vi "PALETTE.vi"   [LabVIEW 2020]
uses:
  Typedefs/Frame Size.ctl
  Typedefs/AOL modes.ctl
  Typedefs/Plane Mode.ctl
  User Interface/Visualisation/Functional Imaging Viewer/SubVIs/Experiment header interface/Typedefs/Header parameters cluster-Live imaging.ctl
  Typedefs/AOL Properties Cluster.ctl
  Global Variables/General Globals.vi
  User Interface/Visualisation/Functional Imaging Viewer/xcontrol/Typedefs/Xctl-XY data type definition.ctl
  User Interface/Visualisation/Functional Imaging Viewer/xcontrol/XGrapher.xctl
  User Interface/Visualisation/Functional Imaging Viewer/xcontrol/Typedefs/Xcrtl-Data format definition.ctl
  User Interface/Visualisation/Functional Imaging Viewer/Typedefs/Get-Set-Clear Control.ctl
  User Interface/Visualisation/Functional Imaging Viewer/xcontrol/Typedefs/Xctrl-ROI type enum.ctl
types:
  T1 = typedef "Get-Set-Clear Control.ctl" = enum16{"Get", "Set", "Clear"}
  T2 = typedef "XGrapher.xctl/Xcrtl-Data format definition.ctl" = cluster{"Plot.Plot Name":string, "Data":T3, "Timeline data":T3, "Type":T4, "Points per cycle":u16, "ROI index":u16}
  T3 = typedef "XGrapher.xctl/Xctl-XY data type definition.ctl" = cluster{"X-Axis values":sgl[], "Y-Axis values (s)":sgl[]}
  T4 = typedef "Xctrl-ROI type enum.ctl" = enum16{"POI", "Mini-scan", "Group"}
  T5 = typedef "Header parameters cluster-Live imaging.ctl" = cluster{"Frame Size":T6, "Field of View":dbl, "Zoom":u16, "X centre":dbl, "Y centre":dbl, "DwellTime (us)":dbl, "AOL Z":dbl, "Wavelength (nm)":dbl, "Laser power (%)":u8, "Pockels":dbl, "Back Apperture":dbl, "PMT 1":dbl, "PMT 2":dbl, "# Averaged Frames":u8, "AOL Mode":T7, "Angle (degrees)":dbl, "Plane Mode":T8, "Video length (sec)":dbl, "Frame rate (fps)":u8, "Fill time (us)":dbl}
  T6 = typedef "Frame Size.ctl" = u16
  T7 = typedef "AOL modes.ctl" = enum16{"Raster", "Structural", "Pointing", "Mini Scan", "Alignment"}
  T8 = typedef "Plane Mode.ctl" = u16
  T9 = typedef "AOL Properties Cluster.ctl" = cluster{"AOD 1 thickness (mm)":dbl, "AOD 2 thickness (mm)":dbl, "AOD 3 thickness (mm)":dbl, "AOD 4 thickness (mm)":dbl, "AOD 5 thickness (mm)":dbl, "AOD 6 thickness (mm)":dbl, "AOD 1-2 separation (mm)":dbl, "AOD 2-3 separation (mm)":dbl, "AOD 3-4 separation (mm)":dbl, "AOD 4-5 separation (mm)":dbl, "AOD 5-6 separation (mm)":dbl, "AOD 1 X Offset":dbl, "AOD 2 X Offset":dbl, "AOD 3 X Offset":dbl, "AOD 4 X Offset":dbl, "AOD 1 Y Offset":dbl, "AOD 2 Y Offset":dbl, "AOD 3 Y Offset":dbl, "AOD 4 Y Offset":dbl, "AOD 1 X Direction":dbl, "AOD 2 X Direction":dbl, "AOD 3 X Direction":dbl, "AOD 4 X Direction":dbl, "AOD 1 Y Direction":dbl, "AOD 2 Y Direction":dbl, "AOD 3 Y Direction":dbl, "AOD 4 Y Direction":dbl, "AOD 1 Centre (mm)":dbl, "AOD 2 Centre (mm)":dbl, "AOD 3 Centre (mm)":dbl, "AOD 4 Centre (mm)":dbl, "Timing Offset AOD 1":dbl, "Timing Offset AOD 2":dbl, "Timing Offset AOD 3":dbl, "Timing Offset AOD 4":dbl, "AOD Optical offset 1":dbl, "AOD Optical offset 2":dbl, "AOL aperture (mm)":dbl, "AOL centre wavelength (nm)":dbl, "AOL centre frequency (MHz)":dbl, "Diffraction mode":dbl, "Crystal length (mm)":dbl, "Acoustic velocity (m/s)":dbl, "Pair deflection ratio":dbl, "AOD fill time (us)":dbl, "AOD Ord. Refractive index":dbl, "AOD ExtraOrd. Refractive index":dbl}
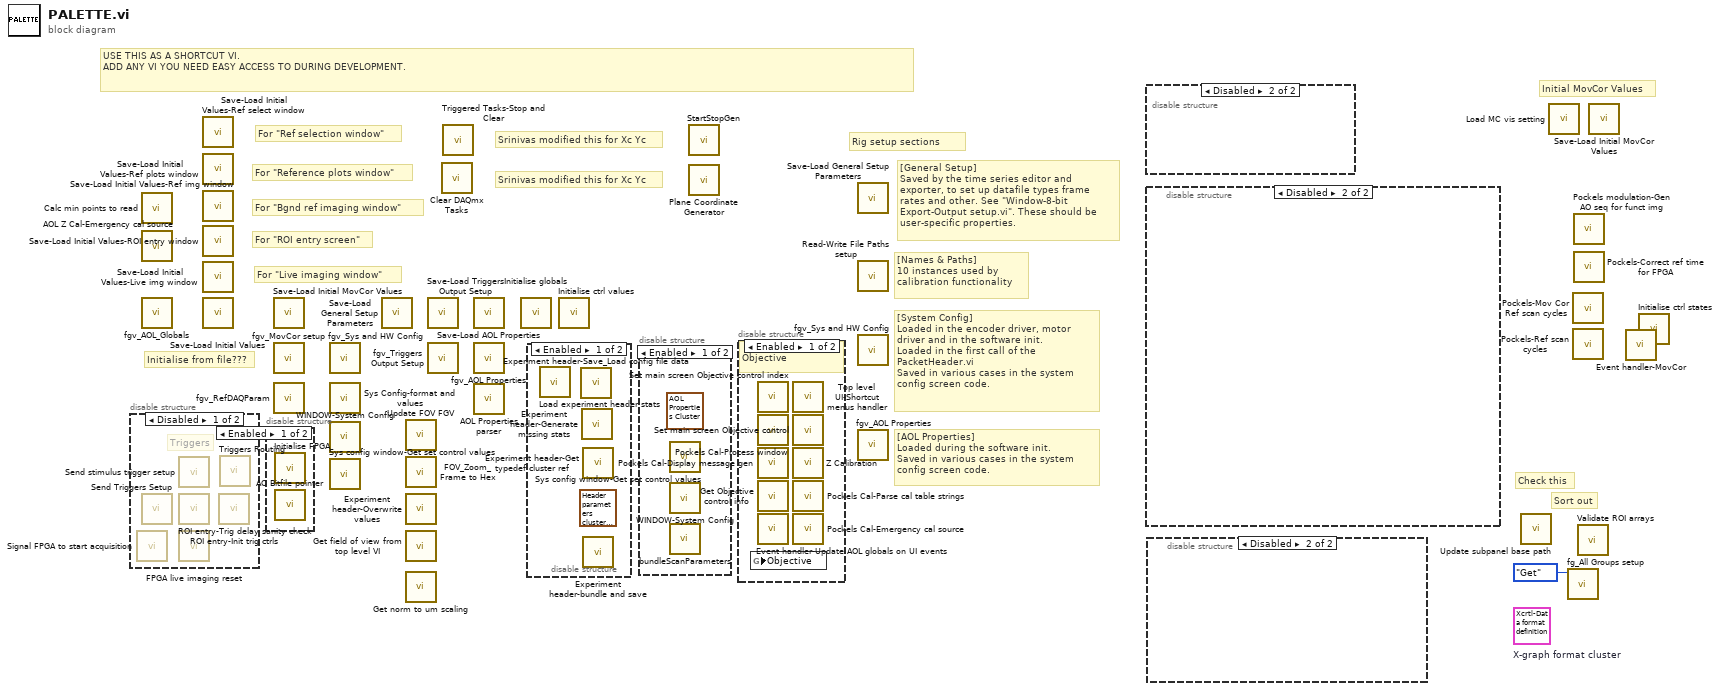
[diagram p0: block diagram]
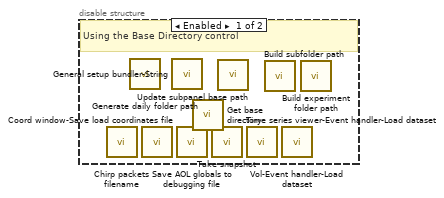
[diagram p2: hidden frame]
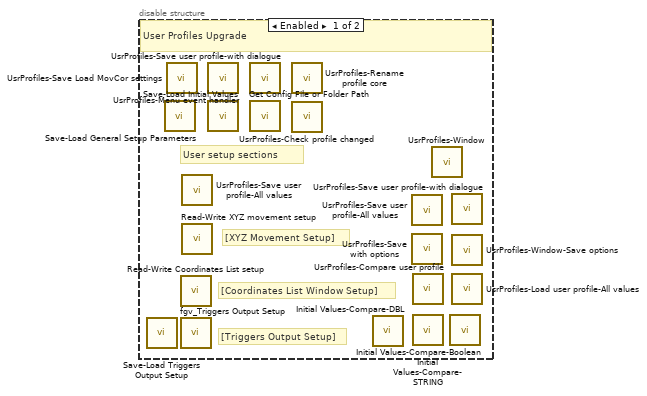
[diagram p3: hidden frame]
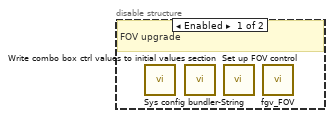
[diagram p4: hidden frame]
diagram:
  (unwired) T2 {"Plot.Plot Name"="", "Data"={"X-Axis values"=[], "Y-Axis values (s)"=[]}, "Timeline data"={"X-Axis values"=[], "Y-Axis values (s)"=[]}, "Type"=enum."POI", "Points per cycle"=0, "ROI index"=0}  # X-graph format cluster
  # "Initial MovCor Values"
  # "Sort out"
  # "Check this"
  # "[AOL Properties]\nLoaded during the software init.\nSaved in various cases in the system config screen code."
  # "[System Config]\nLoaded in the encoder driver, motor driver and in the software init.\nLoaded in the first call of the PacketHeader.vi\nSaved in various cases in the system config screen code."
  # "[Names & Paths]\n10 instances used by calibration functionality"
  # "[General Setup]\nSaved by the time series editor and exporter, to set up datafile types frame rates and other. See \"Window-8-bit Export-Output setup.vi\". These should be user-specific properties."
  # "Rig setup sections"
  # "Srinivas modified this for Xc Yc"
  # "Srinivas modified this for Xc Yc"
  # "For \"Ref selection window\""
  # "For \"Reference plots window\""
  # "For \"Bgnd ref imaging window\""
  # "For \"ROI entry screen\""
  # "For \"Live imaging window\""
  # "Initialise from file???"
  # "USE THIS AS A SHORTCUT VI.\nADD ANY VI YOU NEED EASY ACCESS TO DURING DEVELOPMENT."
  n1 = disable-structure shown="Disabled" {
    frame Disabled {
      # "Triggers"
      n2 = call "Signal FPGA to start acquisition.vi"() -> ()  [unwired: 10 in, 2 out]
      n3 = call "Send Triggers Setup.vi"() -> ()  [unwired: 10 in, 2 out]
      n4 = call "Send stimulus trigger setup.vi"() -> ()  [unwired: 10 in, 2 out]
      n5 = call "ROI entry-Trig delay sanity check.vi"() -> ()  [unwired: 10 in, 2 out]
      n6 = call "FPGA live imaging reset.vi"() -> ()  [unwired: 11 in, 1 out]
      n7 = call "ROI entry-Init trig ctrls.vi"() -> ()  [unwired: 11 in, 1 out]
      n8 = call "Triggers Routing.vi"() -> ()  [unwired: 11 in, 1 out]
    }
    frame Enabled {
    }
  }
  n9 = call "Calc min points to read.vi"() -> ()  [unwired: 3 in, 3 out]
  n10 = call "AOL Z Cal-Emergency cal source.vi"() -> ()  [unwired: 9 in, 3 out]
  n11 = call "fgv_AOL_Globals.vi"() -> ()  [unwired: 10 in, 2 out]
  n12 = call "Save-Load Initial Values-Ref select window.vi"() -> ()  [unwired: 11 in, 1 out]
  n13 = call "Save-Load Initial Values-Ref plots window.vi"() -> ()  [unwired: 11 in, 1 out]
  n14 = call "Save-Load Initial Values-Ref img window.vi"() -> ()  [unwired: 11 in, 1 out]
  n15 = call "Save-Load Initial Values-ROI entry window.vi"() -> ()  [unwired: 11 in, 1 out]
  n16 = call "Save-Load Initial Values-Live img window.vi"() -> ()  [unwired: 11 in, 1 out]
  n17 = call "Save-Load Initial Values.vi"() -> ()  [unwired: 11 in, 1 out]
  n18 = disable-structure shown="Enabled" {
    frame Enabled {
      n19 = call "Initialise FPGA.vi"() -> ()  [unwired: 10 in, 2 out]
      n20 = call "AC Bitfile pointer.vi"() -> ()  [unwired: 10 in, 2 out]
    }
    frame Disabled {
    }
  }
  n21 = call "Save-Load Initial MovCor Values.vi"() -> ()  [unwired: 11 in, 1 out]
  n22 = call "fgv_MovCor setup.vi"() -> ()  [unwired: 10 in, 2 out]
  n23 = call "fgv_RefDAQParam.vi"() -> ()  [unwired: 10 in, 2 out]
  n24 = call "fgv_Sys and HW Config.vi"() -> ()  [unwired: 9 in, 3 out]
  n25 = call "Sys Config-format and values.vi"() -> ()  [unwired: 13 in, 7 out]
  n26 = call "WINDOW-System Config.vi"() -> ()  [unwired: 12 in]
  n27 = call "Sys config window-Get set control values.vi"() -> ()  [unwired: 10 in, 2 out]
  n28 = call "Save-Load General Setup Parameters.vi"() -> ()  [unwired: 11 in, 1 out]
  n29 = call "Update FOV FGV.vi"() -> ()  [unwired: 11 in, 1 out]
  n30 = call "FOV_Zoom_Frame to Hex.vi"() -> ()  [unwired: 11 in, 1 out]
  n31 = call "Experiment header-Overwrite values.vi"() -> ()  [unwired: 10 in, 2 out]
  n32 = call "Get field of view from top level VI.vi"() -> ()  [unwired: 11 in, 1 out]
  n33 = call "Get norm to um scaling .vi"() -> ()  [unwired: 8 in, 4 out]
  n34 = call "Save-Load Triggers Output Setup.vi"() -> ()  [unwired: 9 in, 3 out]
  n35 = call "fgv_Triggers Output Setup.vi"() -> ()  [unwired: 9 in, 3 out]
  n36 = call "Clear DAQmx Tasks.vi"() -> ()  [unwired: 11 in, 1 out]
  n37 = call "Triggered Tasks-Stop and Clear.vi"() -> ()  [unwired: 11 in, 1 out]
  n38 = call "Save-Load AOL Properties.vi"() -> ()  [unwired: 10 in, 2 out]
  n39 = call "fgv_AOL Properties.vi"() -> ()  [unwired: 10 in, 2 out]
  n40 = call "AOL Properties parser.vi"() -> ()  [unwired: 14 in, 6 out]
  n41 = call "Initialise globals.vi"() -> ()  [unwired: 11 in, 1 out]
  n42 = disable-structure shown="Enabled" {
    frame Enabled {
      (unwired) T5 {"Frame Size"=200, "Field of View"=0.0, "Zoom"=0, "X centre"=0.0, "Y centre"=0.0, "DwellTime (us)"=0.0, "AOL Z"=0.0, "Wavelength (nm)"=0.0, "Laser power (%)"=0, "Pockels"=0.0, "Back Apperture"=0.0, "PMT 1"=0.0, "PMT 2"=0.0, "# Averaged Frames"=0, "AOL Mode"=enum."Raster", "Angle (degrees)"=0.0, "Plane Mode"=0, "Video length (sec)"=0.0, "Frame rate (fps)"=0, "Fill time (us)"=0.0} ("Header parameters-Live imaging")
      n43 = call "Load experiment header stats.vi"() -> ()  [unwired: 10 in, 2 out]
      n44 = call "Experiment header-Save_Load config file data.vi"() -> ()  [unwired: 10 in, 2 out]
      n45 = call "Experiment header-Generate missing stats.vi"() -> ()  [unwired: 9 in, 3 out]
      n46 = call "Experiment header-Get typedef cluster ref.vi"() -> ()  [unwired: 8 in, 4 out]
      n47 = call "Experiment header-bundle and save.vi"() -> ()  [unwired: 11 in, 1 out]
    }
    frame Disabled {
    }
  }
  n48 = call "Initialise ctrl values.vi"() -> ()  [unwired: 11 in, 1 out]
  n49 = disable-structure shown="Enabled" {
    frame Enabled {
      (unwired) T9 {"AOD 1 thickness (mm)"=118.0, "AOD 2 thickness (mm)"=115.0, "AOD 3 thickness (mm)"=110.0, "AOD 4 thickness (mm)"=135.0, "AOD 5 thickness (mm)"=135.0, "AOD 6 thickness (mm)"=135.0, "AOD 1-2 separation (mm)"=15.0, "AOD 2-3 separation (mm)"=15.0, "AOD 3-4 separation (mm)"=15.0, "AOD 4-5 separation (mm)"=15.0, "AOD 5-6 separation (mm)"=15.0, "AOD 1 X Offset"=15.0, "AOD 2 X Offset"=1.0, "AOD 3 X Offset"=1.0, "AOD 4 X Offset"=1.0, "AOD 1 Y Offset"=1.0, "AOD 2 Y Offset"=1.0, "AOD 3 Y Offset"=1.0, "AOD 4 Y Offset"=0.0, "AOD 1 X Direction"=0.0, "AOD 2 X Direction"=0.0, "AOD 3 X Direction"=0.0, "AOD 4 X Direction"=0.0, "AOD 1 Y Direction"=0.0, "AOD 2 Y Direction"=0.0, "AOD 3 Y Direction"=0.0023, "AOD 4 Y Direction"=0.0046, "AOD 1 Centre (mm)"=15.0, "AOD 2 Centre (mm)"=50.0, "AOD 3 Centre (mm)"=50.0, "AOD 4 Centre (mm)"=50.0, "Timing Offset AOD 1"=0.0, "Timing Offset AOD 2"=0.0, "Timing Offset AOD 3"=0.0, "Timing Offset AOD 4"=0.0, "AOD Optical offset 1"=0.0, "AOD Optical offset 2"=0.0, "AOL aperture (mm)"=0.0, "AOL centre wavelength (nm)"=0.0, "AOL centre frequency (MHz)"=0.0, "Diffraction mode"=0.0, "Crystal length (mm)"=0.0, "Acoustic velocity (m/s)"=0.0, "Pair deflection ratio"=0.0, "AOD fill time (us)"=0.0, "AOD Ord. Refractive index"=0.0, "AOD ExtraOrd. Refractive index"=2.22} ("AOL Properties")
      n50 = call "Sys config window-Get set control values.vi"() -> ()  [unwired: 10 in, 2 out]
      n51 = call "WINDOW-System Config.vi"() -> ()  [unwired: 12 in]
      n52 = call "bundleScanParameters.vi"() -> ()  [unwired: 5 in, 7 out]
    }
    frame Disabled {
    }
  }
  n53 = call "StartStopGen.vi"() -> ()  [unwired: 11 in, 1 out]
  n54 = call "Plane Coordinate Generator.vi"() -> ()  [unwired: 10 in, 2 out]
  n55 = disable-structure shown="Enabled" {
    frame Enabled {
      # "Objective"
      n56 = global read "General Globals.vi" "Objective"() -> ()  [unwired: 1 in]
      n57 = call "Set main screen Objective control index.vi"() -> ()  [unwired: 10 in, 2 out]
      n58 = call "Pockels Cal-Process window.vi"() -> ()  [unwired: 10 in, 2 out]
      n59 = call "Pockels Cal-Display message gen.vi"() -> ()  [unwired: 11 in, 1 out]
      n60 = call "Get Objective control info.vi"() -> ()  [unwired: 7 in, 5 out]
      n61 = call "Event handler-Update AOL globals on UI events.vi"() -> ()  [unwired: 11 in, 1 out]
      n62 = call "Top level UI-Shortcut menus handler.vi"() -> ()  [unwired: 12 in]
      n63 = call "Set main screen Objective control.vi"() -> ()  [unwired: 11 in, 1 out]
      n64 = call "Z Calibration.vi"() -> ()  [unwired: 8 in, 4 out]
      n65 = call "Pockels Cal-Parse cal table strings.vi"() -> ()  [unwired: 6 in, 6 out]
      n66 = call "Pockels Cal-Emergency cal source.vi"() -> ()  [unwired: 11 in, 1 out]
    }
    frame Disabled {
    }
  }
  n67 = call "Save-Load General Setup Parameters.vi"() -> ()  [unwired: 11 in, 1 out]
  n68 = call "Read-Write File Paths setup.vi"() -> ()  [unwired: 11 in, 1 out]
  n69 = call "fgv_Sys and HW Config.vi"() -> ()  [unwired: 9 in, 3 out]
  n70 = call "fgv_AOL Properties.vi"() -> ()  [unwired: 10 in, 2 out]
  n71 = disable-structure shown="Disabled" {
    frame Enabled {
      # "FOV upgrade"
      n72 = call "Sys config bundler-String.vi"() -> ()  [unwired: 9 in, 3 out]
      n73 = call "Write combo box ctrl values to initial values section.vi"() -> ()  [unwired: 11 in, 1 out]
      n74 = call "Set up FOV control.vi"() -> ()  [unwired: 11 in, 1 out]
      n75 = call "fgv_FOV.vi"() -> ()  [unwired: 8 in, 4 out]
    }
    frame Disabled {
    }
  }
  n76 = disable-structure shown="Disabled" {
    frame Enabled {
      # "[Triggers Output Setup]"
      # "[Coordinates List Window Setup]"
      # "[XYZ Movement Setup]"
      # "User setup sections"
      # "User Profiles Upgrade"
      n77 = call "Save-Load Triggers Output Setup.vi"() -> ()  [unwired: 9 in, 3 out]
      n78 = call "Save-Load General Setup Parameters.vi"() -> ()  [unwired: 11 in, 1 out]
      n79 = call "UsrProfiles-Save Load MovCor settings.vi"() -> ()  [unwired: 11 in, 1 out]
      n80 = call "Read-Write Coordinates List setup.vi"() -> ()  [unwired: 11 in, 1 out]
      n81 = call "fgv_Triggers Output Setup.vi"() -> ()  [unwired: 9 in, 3 out]
      n82 = call "UsrProfiles-Save user profile-All values.vi"() -> ()  [unwired: 11 in, 1 out]
      n83 = call "Read-Write XYZ movement setup.vi"() -> ()  [unwired: 11 in, 1 out]
      n84 = call "UsrProfiles-Menu event handler.vi"() -> ()  [unwired: 12 in]
      n85 = call "Save-Load Initial Values.vi"() -> ()  [unwired: 11 in, 1 out]
      n86 = call "UsrProfiles-Save user profile-with dialogue.vi"() -> ()  [unwired: 12 in]
      n87 = call "Get Config File or Folder Path.vi"() -> ()  [unwired: 9 in, 3 out]
      n88 = call "UsrProfiles-Rename profile core.vi"() -> ()  [unwired: 8 in, 4 out]
      n89 = call "UsrProfiles-Check profile changed.vi"() -> ()  [unwired: 10 in, 2 out]
      n90 = call "Initial Values-Compare-DBL.vi"() -> ()  [unwired: 7 in, 5 out]
      n91 = call "UsrProfiles-Save user profile-All values.vi"() -> ()  [unwired: 11 in, 1 out]
      n92 = call "UsrProfiles-Save with options.vi"() -> ()  [unwired: 11 in, 1 out]
      n93 = call "UsrProfiles-Compare user profile.vi"() -> ()  [unwired: 10 in, 2 out]
      n94 = call "Initial Values-Compare-STRING.vi"() -> ()  [unwired: 7 in, 5 out]
      n95 = call "UsrProfiles-Window.vi"() -> ()  [unwired: 10 in, 2 out]
      n96 = call "Initial Values-Compare-Boolean.vi"() -> ()  [unwired: 7 in, 5 out]
      n97 = call "UsrProfiles-Save user profile-with dialogue.vi"() -> ()  [unwired: 12 in]
      n98 = call "UsrProfiles-Window-Save options.vi"() -> ()  [unwired: 10 in, 2 out]
      n99 = call "UsrProfiles-Load user profile-All values.vi"() -> ()  [unwired: 11 in, 1 out]
    }
    frame Disabled {
    }
  }
  n100 = disable-structure shown="Disabled" {
    frame Enabled {
      # "Using the Base Directory control"
      n101 = call "Chirp packets filename.vi"() -> ()  [unwired: 10 in, 2 out]
      n102 = call "Generate daily folder path.vi"() -> ()  [unwired: 11 in, 1 out]
      n103 = call "Coord window-Save load coordinates file.vi"() -> ()  [unwired: 11 in, 1 out]
      n104 = call "General setup bundler-String.vi"() -> ()  [unwired: 10 in, 2 out]
      n105 = call "Save AOL globals to debugging file.vi"() -> ()  [unwired: 12 in]
      n106 = call "Get base directory.vi"() -> ()  [unwired: 3 in, 1 out]
      n107 = call "Take snapshot.vi"() -> ()  [unwired: 12 in]
      n108 = call "Update subpanel base path.vi"() -> ()  [unwired: 11 in, 1 out]
      n109 = call "Time series viewer-Event handler-Load dataset.vi"() -> ()  [unwired: 12 in]
      n110 = call "Build subfolder path.vi"() -> ()  [unwired: 10 in, 2 out]
      n111 = call "Vol-Event handler-Load dataset.vi"() -> ()  [unwired: 12 in]
      n112 = call "Build experiment folder path.vi"() -> ()  [unwired: 10 in, 2 out]
    }
    frame Disabled {
    }
  }
  n113 = call "Update subpanel base path.vi"() -> ()  [unwired: 11 in, 1 out]
  n114 = call "Load MC vis setting.vi"() -> ()  [unwired: 10 in, 2 out]
  n115 = call "fg_All Groups setup.vi"("Function"=Get-Set-Clear_Control."Get") -> ()  [unwired: 9 in, 2 out]
  n116 = call "Pockels-Mov Cor Ref scan cycles.vi"() -> ()  [unwired: 11 in, 1 out]
  n117 = call "Pockels-Ref scan cycles.vi"() -> ()  [unwired: 10 in, 2 out]
  n118 = call "Pockels modulation-Gen AO seq for funct img.vi"() -> ()  [unwired: 8 in, 4 out]
  n119 = call "Pockels-Correct ref time for FPGA.vi"() -> ()  [unwired: 10 in, 2 out]
  n120 = call "Validate ROI arrays.vi"() -> ()  [unwired: 10 in, 2 out]
  n121 = call "Save-Load Initial MovCor Values.vi"() -> ()  [unwired: 11 in, 1 out]
  n122 = call "Event handler-MovCor.vi"() -> ()  [unwired: 11 in, 1 out]
  n123 = call "Initialise ctrl states.vi"() -> ()  [unwired: 11 in, 1 out]
